vi "Mask Actions.vi"(6 "AutoAlign Timeout (1 s)":dbl=1.0, 7 "Alignment Type (8: None)":i32(ring)=8 items=["EYEAMI", "EYECMI", "EYENRZ", "FANWidth", "FAPeriod", "FAPWidth", "FYNWidth", "FYPWidth", "None", "NWidth", "PWidth", "TMax", "TMin"], 8 "error in (no error)":errorcluster, 9 "Filename":string, 10 "Actions (0: Align)":i32(ring) items=["Align", "Create AutoMask", "Save AutoMask", "Load Mask", "Delete Mask", "Invert Mask", "Revert Mask"], 11 "VISA resource name":refnum<visa-resource-name>) -> (0 "error out":errorcluster, 3 "VISA resource name out":refnum<visa-resource-name>)   [LabVIEW 2020, in "Agilent 90000 Series.lvlib"]
doc: "Performs various mask and automask actions."
uses:
  Agilent 90000 Series.lvlib
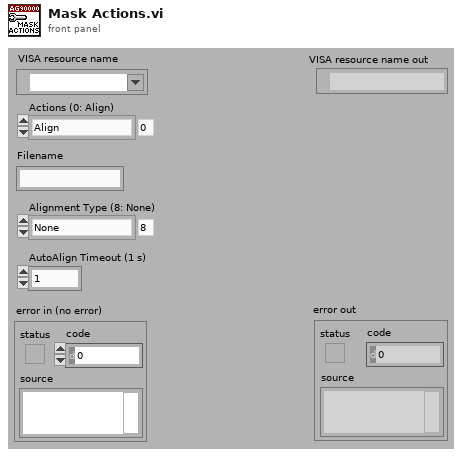
[diagram p1: front panel]
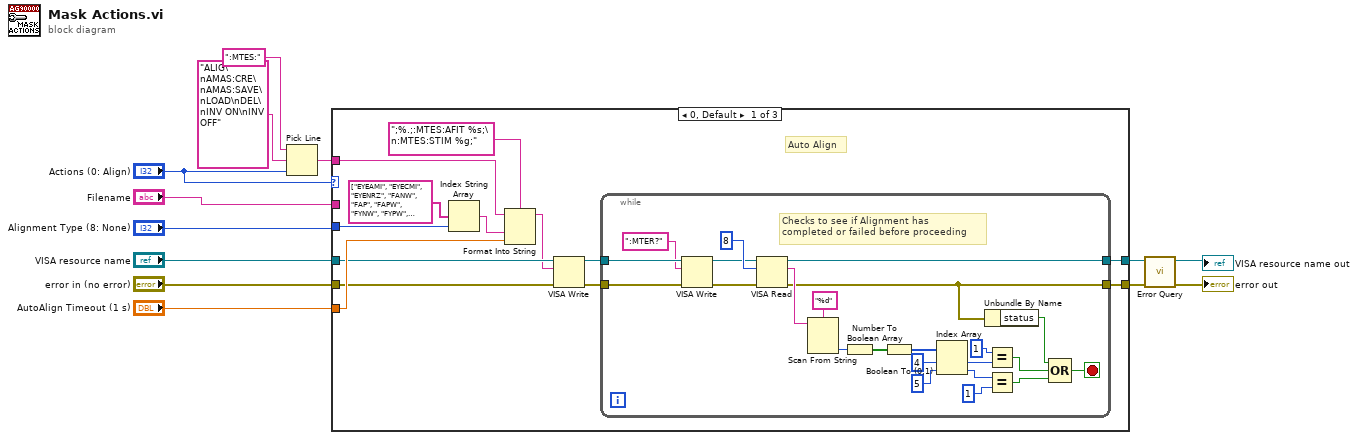
[diagram p0: block diagram]
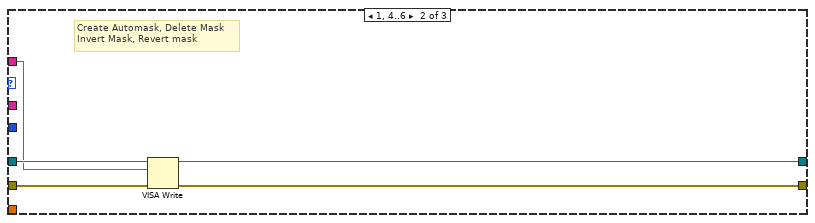
[diagram p2: hidden frame]
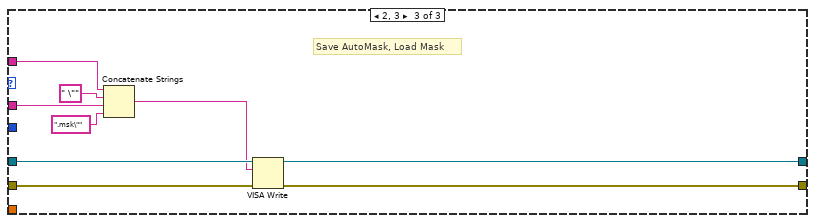
[diagram p3: hidden frame]
diagram:
  n1 = Pick Line(string ("")=":MTES:", multi-line string="ALIG\nAMAS:CRE\nAMAS:SAVE\nLOAD\nDEL\nINV ON\nINV OFF", line index="Actions (0: Align)") -> (output string=w9:string)
  n2 = case shown="0, Default" "Actions (0: Align)" {
    tunnel: "Filename" -> [_ _ w63]
    tunnel: "Alignment Type (8: None)" -> [w23 _ _]
    tunnel: "AutoAlign Timeout (1 s)" -> [w22 _ _]
    tunnel: w9 -> [w21 w52 w60]
    tunnel: "VISA resource name" -> [w20 w54 w59]
    tunnel: "error in (no error)" -> [w19 w53 w58]
    tunnel: [w15 w51 w57] -> w6
    tunnel: [w14 w50 w56] -> w5
    frame 0, Default {
      # "Auto Align"
      n3 = Index String Array(1:w23, 2:string[] ["EYEAMI", "EYECMI", "EYENRZ", "FANW", "FAP", "FAPW", "FYNW", "FYPW", "NONE", "NWID", "PWID", "TMAX", "TMIN"] ("string array")) -> (0:w24:string)  [unwired: 1 out]
      n4 = Format Into String(format string=";%.;:MTES:AFIT %s;\n:MTES:STIM %g;", initial string=w21, w24, w22) -> (resulting string=w18:string)  [unwired: 1 in, 1 out]
      n5 = VISA Write(VISA resource name=w20, write buffer=w18, error in (no error)=w19) -> (VISA resource name out=w17:refnum<visa-resource-name>, error out=w16:errorcluster)  [unwired: 1 out]
      n6 = while {
        tunnel: w17 -> [w31]
        tunnel: w16 -> [w30]
        tunnel: [w42] -> w15
        tunnel: [w35] -> w14
        stop <- w36 stop-if-true
        # "Checks to see if Alignment has\ncompleted or failed before proceeding"
        n7 = VISA Write(VISA resource name=w31, write buffer=":MTER?", error in (no error)=w30) -> (VISA resource name out=w29:refnum<visa-resource-name>, error out=w28:errorcluster)  [unwired: 1 out]
        n8 = VISA Read(VISA resource name=w29, byte count=u32 8, error in (no error)=w28) -> (VISA resource name out=w42:refnum<visa-resource-name>, read buffer=w48:string, error out=w35:errorcluster)  [unwired: 1 out]
        n9 = Scan From String(format string="%d", input string=w48) -> (output 1=w45:i32)  [unwired: 2 in, 4 out]
        n10 = Number To Boolean Array(number=w45) -> (Boolean array=w46:bool[])
        n11 = Boolean To (0,1)(Boolean=w46) -> (0, 1=w44:i16[])
        n12 = Index Array(array=w44, index #1=4 ("index"), index #2=5 ("index")) -> (element #1=w40:i16, element #2=w38:i16)
        n13 = Unbundle By Name(w35) -> ("status"=w32:bool)
        n14 = Equal?(x=i16 1 ("y"), y=w40) -> (x = y?=w33:bool)
        n15 = Equal?(x=w38, y=i16 1) -> (x = y?=w34:bool)
        n16 = Compound Arithmetic op=OR(w32, w33, w34) -> (w36:bool)
      }
    }
    frame 1, 4..6 {
      # "Create Automask, Delete Mask\nInvert Mask, Revert mask"
      n17 = VISA Write(VISA resource name=w54, write buffer=w52, error in (no error)=w53) -> (VISA resource name out=w51:refnum<visa-resource-name>, error out=w50:errorcluster)  [unwired: 1 out]
    }
    frame 2, 3 {
      # "Save AutoMask, Load Mask"
      n18 = Concatenate Strings(w60, " \"" ("string"), w63, ".msk\"" ("string")) -> (w55:string)
      n19 = VISA Write(VISA resource name=w59, write buffer=w55, error in (no error)=w58) -> (VISA resource name out=w57:refnum<visa-resource-name>, error out=w56:errorcluster)  [unwired: 1 out]
    }
  }
  n20 = call "Error Query.vi"("error in (no error)"=w5, "VISA resource name"=w6) -> ("error out"=→"error out":errorcluster, "VISA resource name out"=→"VISA resource name out":refnum<visa-resource-name>)  [unwired: 8 out]
